vi "NTLogger.vi"(8 "error in (no error)":errorcluster, 11 "occurrence":refnum<k4>) -> ()   [LabVIEW 2015]
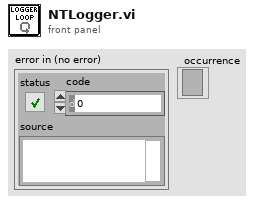
[diagram p1: front panel]
types:
  T1 = enum16{"open", "replace", "create", "open or create", "replace or create", "replace or create with confirmation"}
  T2 = typedef "WPI_DriverStationRobotMode2.ctl" = enum16{"Autonomous Disabled", "Autonomous Enabled", "Teleop Disabled", "Teleop Enabled", "Disconnected", "Finish", "Test Disabled", "Test Enabled", "Emergency Stopped"}
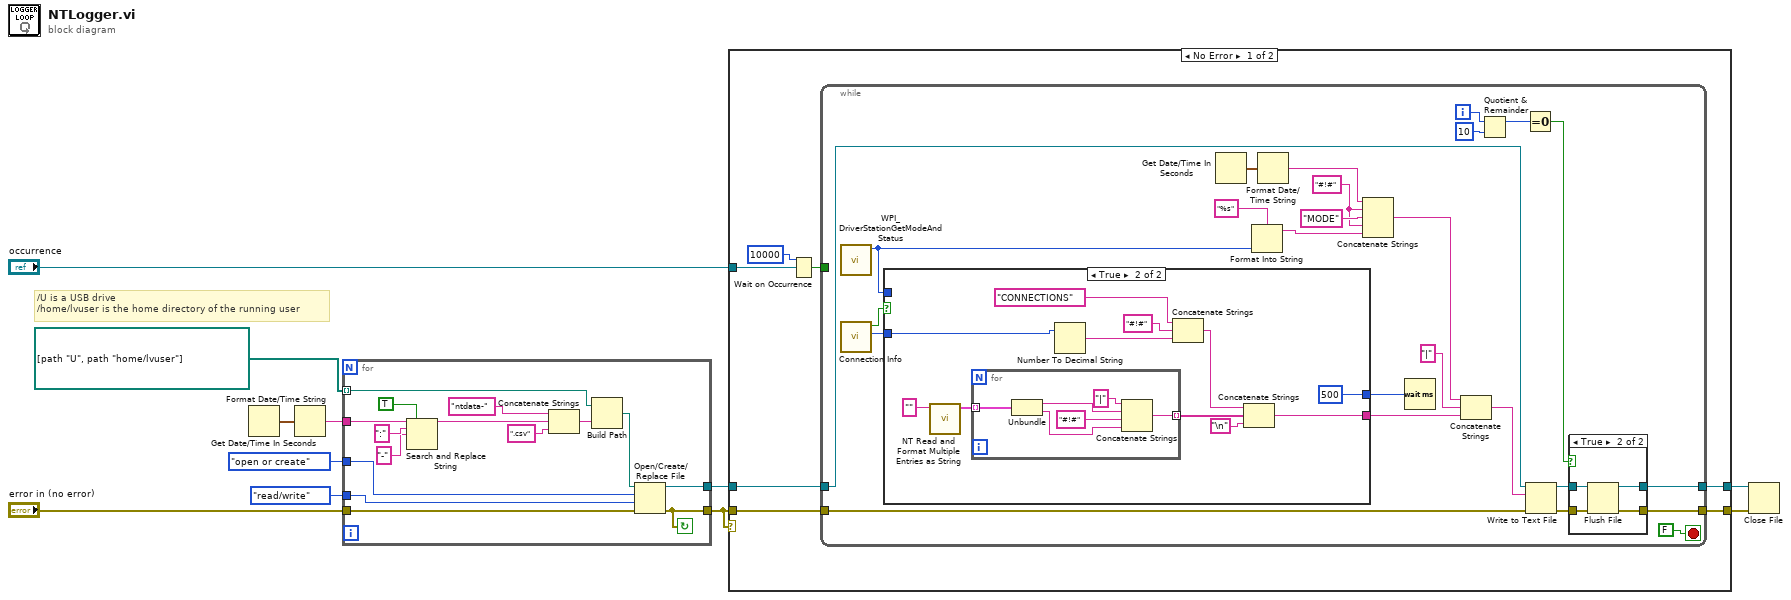
[diagram p0: block diagram]
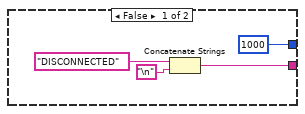
[diagram p3: hidden frame]
diagram:
  # "/U is a USB drive\n/home/lvuser is the home directory of the running user"
  n1 = Get Date/Time In Seconds() -> (seconds since 1Jan1904=w5:timestamp)
  n2 = Format Date/Time String(seconds (now)=w5) -> (date/time string=w4:string)  [unwired: 2 in]
  n3 = for {
    tunnel: [w26] -> w3
    tunnel: T1."open or create" ("operation (0:open)") -> [w24]
    tunnel: enum16{"read/write", "read-only", "write-only"}."read/write" ("access (0:read/write)") -> [w23]
    tunnel: "error in (no error)" -> [w25]
    tunnel: [w21] -> w2
    tunnel: path[] [path "U:/", path "/home/lvuser"] -> [w22] mode=indexing
    tunnel: w4 -> [w14]
    stop <- w21 continue-if-true
    n4 = Search and Replace String(replace all?=TRUE ("replace all? (F)"), input string=w14, search string=":", replace string="-" ("replace string (\"\")")) -> (result string=w13:string)  [unwired: 4 in, 3 out]
    n5 = Concatenate Strings("ntdata-" ("string"), w13, ".csv" ("string")) -> (w12:string)
    n6 = Build Path(base path=w22, name or relative path=w12) -> (appended path=w18:path)
    n7 = Open/Create/Replace File(file path (use dialog)=w18, error in=w25, operation (0:open)=w24, access (0:read/write)=w23) -> (refnum out=w26:refnum<file>, error out=w21:errorcluster)  [unwired: 2 in, 1 out]
  }
  n8 = case shown="No Error" w2 {
    tunnel: [w33 w87] -> w8
    tunnel: [w32 w86] -> w7
    tunnel: w3 -> [w31 w87]
    tunnel: w2 -> [w30 w86]
    tunnel: "occurrence" -> [w29 _]
    frame No Error {
      n9 = Wait on Occurrence(2:w29, 3:10000 ("ms timeout (-1)")) -> (0:w28:bool)  [unwired: 1 in]
      n10 = while {
        tunnel: w31 -> [w56]
        tunnel: w30 -> [w57]
        tunnel: [w39] -> w33
        tunnel: [w40] -> w32
        tunnel: w28 -> [_]
        i -> [w38]
        stop <- FALSE stop-if-true
        w44 = "#!#" ("string")
        n11 = call <vilib>:"WPI_DriverStationGetModeAndStatus.vi"() -> ("Robot Mode"=w52:T2)  [unwired: 10 in, 1 out]
        n12 = call <vilib>:"Connection Info.vi"() -> ("Connection Count"=w58:i32, "Connected"=w46:bool)  [unwired: 10 in]
        n13 = case shown="True" w46 {
          tunnel: w58 -> [_ w77]
          tunnel: [w67 w76] -> w50
          tunnel: w52 -> [_ _]
          tunnel: [u32 1000 ("milliseconds to wait") u32 500 ("milliseconds to wait")] -> w34
          frame False {
            n14 = Concatenate Strings("DISCONNECTED" ("string"), "\n") -> (w67:string)
          }
          frame True {
            n15 = call <vilib>:"NT Read and Format Multiple Entries as String.vi"("Name Pattern"="") -> ("Formatted Strings"=w79:cluster{"Name":string, "Value":string}[])  [unwired: 9 in, 1 out]
            n16 = for {
              tunnel: w79 -> [w85] mode=indexing
              tunnel: [w81] -> w72 mode=indexing
              n17 = Unbundle(w85) -> ("Name"=w84:string, "Value"=w83:string)
              n18 = Concatenate Strings("|" ("string"), w84, "#!#" ("string"), w83) -> (w81:string)
            }
            n19 = Number To Decimal String(number=w77) -> (decimal integer string=w74:string)  [unwired: 1 in]
            n20 = Concatenate Strings("CONNECTIONS" ("string"), "#!#" ("string"), w74) -> (w75:string)
            n21 = Concatenate Strings(w75, w72, "\n") -> (w76:string)
          }
        }
        n22 = Get Date/Time In Seconds() -> (seconds since 1Jan1904=w45:timestamp)
        n23 = Format Into String(format string="%s", w52) -> (resulting string=w55:string)  [unwired: 2 in, 1 out]
        n24 = Format Date/Time String(seconds (now)=w45) -> (date/time string=w43:string)  [unwired: 2 in]
        n25 = Concatenate Strings(w43, w44, "MODE" ("string"), w44, w55) -> (w48:string)
        n26 = Wait (ms)(milliseconds to wait=w34) -> ()  [unwired: 1 out]
        n27 = Concatenate Strings(w48, "|" ("string"), w50) -> (w49:string)
        n28 = Quotient & Remainder(x=w38, y=10) -> (x-y*floor(x/y)=w36:i32)  [unwired: 1 out]
        n29 = Equal To 0?(x=w36) -> (x = 0?=w35:bool)
        n30 = Write to Text File(file (use dialog)=w56, text=w49, error in=w57) -> (refnum out=w42:refnum<file>, error out=w41:errorcluster)  [unwired: 1 in, 1 out]
        n31 = case shown="True" w35 {
          tunnel: w42 -> [w60 w64]
          tunnel: w41 -> [w59 w63]
          tunnel: [w59 w62] -> w40
          tunnel: [w60 w61] -> w39
          frame False {
          }
          frame True {
            n32 = Flush File(refnum=w64, error in=w63) -> (refnum out=w61:refnum<file>, error out=w62:errorcluster)
          }
        }
      }
    }
    frame Error {
    }
  }
  n33 = Close File(refnum=w8, error in=w7) -> ()  [unwired: 2 out]
